vi "Destroy User Events.vi"(11 "Logging in":refnum<class "Logging.lvclass">) -> (3 "Logging out":refnum<class "Logging.lvclass">)   [LabVIEW 2020, in "Logging.lvlib" / "Logging.lvclass"]
uses:
  Logging.lvclass
  Logging.lvclass/Logging.ctl
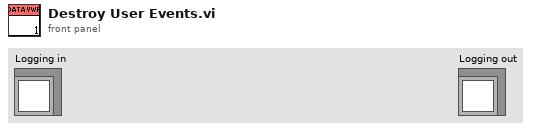
[diagram p1: front panel]
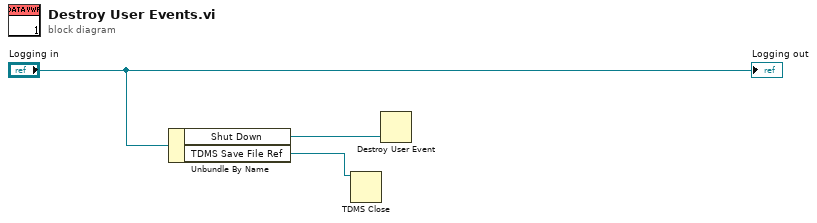
[diagram p0: block diagram]
diagram:
  n1 = Unbundle By Name("Logging in") -> ("Shut Down"=w2:refnum<user-event>, "TDMS Save File Ref"=w1:refnum<k34>)
  n2 = TDMS Close(11:w1) -> ()  [unwired: 1 in, 2 out]
  n3 = Destroy User Event(user event=w2) -> ()  [unwired: 1 in, 1 out]
  "Logging out" <- "Logging in"
